vi "DriveDistance.vi"(1 "Parameter String":string, 2 "Reinit":bool) -> (0 "Increment":bool)   [LabVIEW 2018]
uses:
  dsinstructions.vi
  sensors.vi
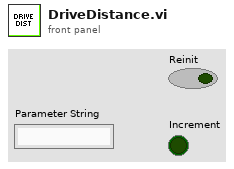
[diagram p1: front panel]
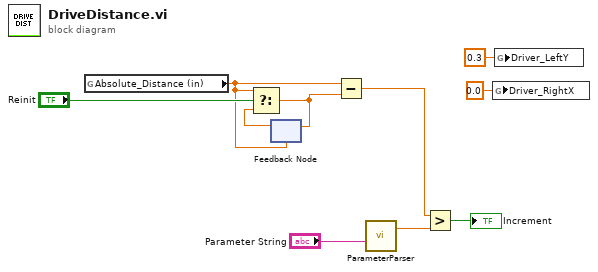
[diagram p0: block diagram]
diagram:
  n1 = global read "sensors.vi" "Absolute_Distance (in)"() -> (w7:dbl)
  n2 = feedback #1(w7) -> (w9:dbl)
  n3 = Select(t=w7, s="Reinit", f=w9) -> (s? t:f=w6:dbl)
  n4 = feedback-in #1(w6) -> ()
  n5 = Subtract(x=w7, y=w6) -> (x-y=w5:dbl)
  n6 = call "ParameterParser.vi"("Parameter String"="Parameter String") -> ("Parameter"=w1:dbl)  [unwired: 1 in, 1 out]
  n7 = Greater?(x=w5, y=w1) -> (0:→"Increment":bool)
  n8 = global write "dsinstructions.vi" "Driver_RightX"(0.0 ("Driver_RightX")) -> ()
  n9 = global write "dsinstructions.vi" "Driver_LeftY"(0.3 ("Driver_LeftY")) -> ()
